vi "PrintNewLineToCLI.vi"(8 "error in (no error)":errorcluster, 11 "CLI in":refnum<class "CLI.lvclass">) -> (0 "error out":errorcluster, 3 "CLI out":refnum<class "CLI.lvclass">)   [LabVIEW 2018]
uses:
  <vilib>/Wiresmith Technology/LabVIEW CLI/CLI Class/CLI.lvclass
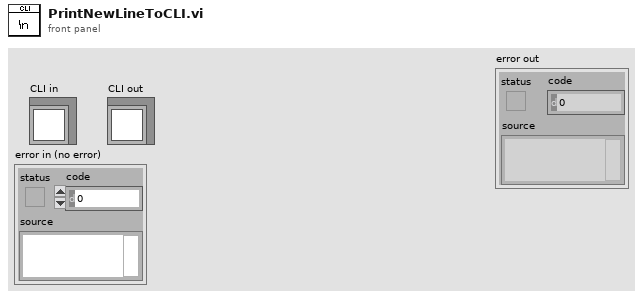
[diagram p1: front panel]
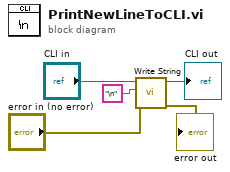
[diagram p0: block diagram]
diagram:
  n1 = call <vilib>:"Write String.vi"("error in (no error)"="error in (no error)", "Text to Write"="\n", "CLI in"="CLI in") -> ("error out"=→"error out":errorcluster, "CLI out"=→"CLI out":refnum<class "CLI.lvclass">)  [unwired: 7 in]
